vi "dfd_Masking Filter Create Specs.vi"(4 "CIC factor":i32, 6 "CIC stage":i32, 8 "ripple specs":T2={"passband"=0.1, "stopband"=40.0, "dB/linear? (T: dB)"=TRUE}, 9 "masking freq specs [Hz]":T1, 11 "masking order":i32) -> (2 "Masking band parameters":T3[](array[typedef])=[{"band specification"=[{"freq"=0.0, "amplitude"=1.0, "weight"=1.0}, {"freq"=0.2, "amplitude"=1.0, "weight"=1.0}], "ripple constraint"=0.0}, {"band specification"=[{"freq"=0.3, "amplitude"=0.0, "weight"=1.0}, {"freq"=0.5, "amplitude"=0.0, "weight"=1.0}], "ripple constraint"=0.0}], 3 "dup masking order":i32)   [LabVIEW 2017, in "NI_DigFilterLicensed.lvlib"]
uses:
  <vilib>/addons/Digital Filter Design/NI_DigFilterLicensed.lvlib
  <vilib>/addons/Digital Filter Design/_Objects.llb/DFD Adv Band Spec.ctl
  <vilib>/addons/Digital Filter Design/_Objects.llb/DFD Filter Ripple Specification (Design).ctl
  <vilib>/addons/Digital Filter Design/_Objects.llb/DFD Filter Frequence Specification (Design).ctl
  <vilib>/Analysis/1siggen.llb/Ramp Pattern by Samples.vi
  <vilib>/addons/Digital Filter Design/NI_DigFilter_Design.lvlib
  <vilib>/Analysis/NI_AALBase.lvlib
panel:
  # "freq"
  # "amplitude"
  # "weight"
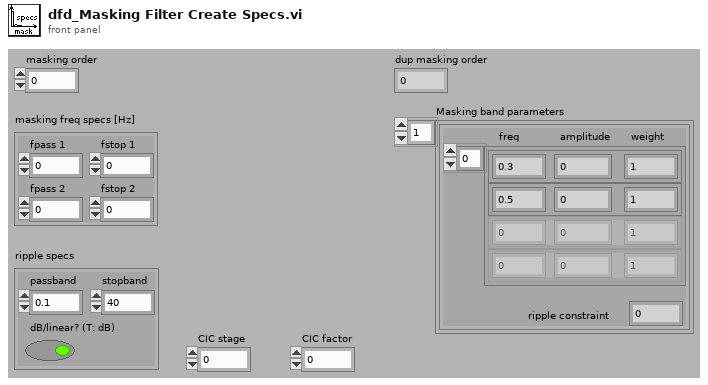
[diagram p1: front panel]
types:
  T1 = typedef "NI_DigFilterLicensed.lvlib/DFD Filter Frequence Specification (Design).ctl" = cluster{"fpass 1":dbl, "fstop 1":dbl, "fpass 2 ":dbl, "fstop 2":dbl}
  T2 = typedef "NI_DigFilterLicensed.lvlib/DFD Filter Ripple Specification (Design).ctl" = cluster{"passband":dbl, "stopband":dbl, "dB/linear? (T: dB)":bool}
  T3 = typedef "NI_DigFilterLicensed.lvlib/DFD Adv Band Spec.ctl" = cluster{"band specification":cluster{"freq":dbl, "amplitude":dbl, "weight":dbl}[], "ripple constraint":dbl}
  T4 = cluster{cluster{dbl, dbl, "Element Data":dbl}[], i32}
  T5 = cluster{cluster{"Element Data":dbl, dbl, dbl}[], i32}
  T6 = cluster{cluster{"Element Data":dbl, dbl, "Element Data":dbl}[], i32}[]
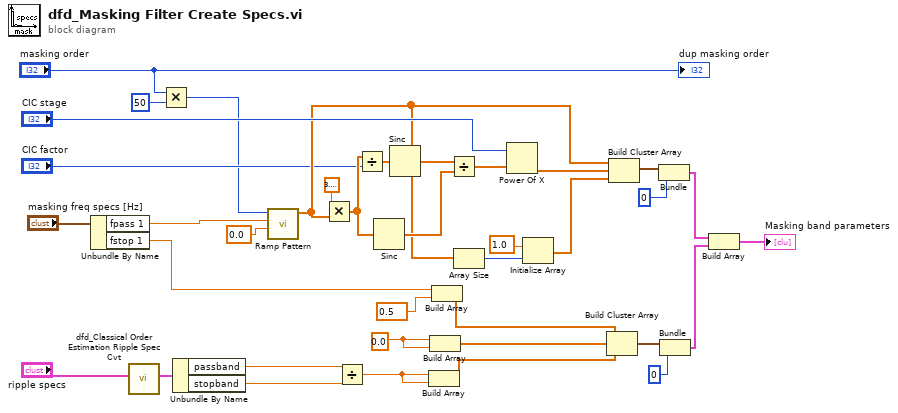
[diagram p0: block diagram]
diagram:
  w27 = 0.0
  n1 = Unbundle By Name("masking freq specs [Hz]") -> ("fpass 1"=w2:dbl, "fstop 1"=w1:dbl)
  n2 = call <vilib>:"dfd_Classical Order Estimation Ripple Spec Cvt.vi"("ripple specs"="ripple specs") -> ("ripple specs (linear)"=w11:T2)  [unwired: 10 out]
  n3 = Multiply(x="masking order", y=50) -> (x*y=w4:i32)
  n4 = Unbundle By Name(w11) -> ("passband"=w10:dbl, "stopband"=w9:dbl)
  n5 = call-poly <vilib>:"Ramp Pattern.vi"("start"=0.0, "end"=w2, "samples"=w4) -> ("Ramp Pattern"=w14:dbl[])  [unwired: 7 in, 1 out]
  n6 = Multiply(x=3.141592653589793, y=w14) -> (x*y=w33:dbl[])
  n7 = Divide(x=w10, y=w9) -> (x/y=w7:dbl)
  n8 = Divide(x=w33, y="CIC factor") -> (x/y=w34:dbl[])
  n9 = Sinc(1:w33) -> (0:w31:dbl[])
  n10 = Sinc(1:w34) -> (0:w32:dbl[])
  n11 = Build Array(w7, w7) -> (w24:dbl[])
  n12 = Build Array(w27, w27) -> (w25:dbl[])
  n13 = Build Array(w1, 0.5 ("Element Data")) -> (w26:dbl[])
  n14 = Divide(x=w32, y=w31) -> (x/y=w30:dbl[])
  n15 = Array Size(array=w14) -> (size(s)=w16:i32)
  n16 = Power Of X(1:w30, 2:"CIC stage") -> (0:w13:dbl[])
  n17 = Initialize Array(1.0 ("Element Data"), w16) -> (w28:dbl[])
  n18 = Build Cluster Array(w26, w25, w24) -> (w19:cluster{"Element Data":dbl, dbl, dbl}[])
  n19 = Build Cluster Array(w14, w13, w28) -> (w22:cluster{dbl, dbl, "Element Data":dbl}[])
  n20 = Bundle(w22, 0) -> (w20:T4)  [unwired: 1 out]
  n21 = Bundle(w19, 0) -> (w17:T5)  [unwired: 1 out]
  n22 = Build Array(w20, w17) -> (→"Masking band parameters":T6)
  "dup masking order" <- "masking order"
